vi "Stop Core.vi"(10 "final error code":i32, 11 "Car Wash Controller in":refnum<class "Car Wash Controller.lvclass">) -> (3 "Car Wash Controller out":refnum<class "Car Wash Controller.lvclass">)   [LabVIEW 2019, in "Car Wash Controller.lvlib" / "Car Wash Controller.lvclass"]
doc: "(<B>Filename</B>: Actor Framework.lvlib:Actor.lvclass:Stop Core.vi)\n\nDefines what the actor does before it stops. Use the <B>final error code</B> input to determine whether the actor shut down in response to an error.\n\nBy default, this method passes the Stop message along to all auto-stop nested actors. A descendant class may override this method to define additional behavior, such as shutting down any processes the actor initiated in its override of the Actor Core method."
uses:
  Car Wash Controller.lvclass
  Car Wash Controller.lvclass/Car Wash Controller.ctl
  <vilib>/ActorFramework/Actor/Actor.lvclass
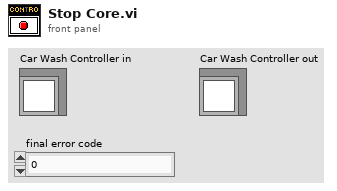
[diagram p1: front panel]
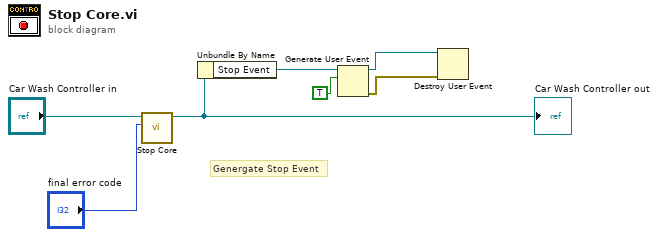
[diagram p0: block diagram]
diagram:
  # "Genergate Stop Event"
  n1 = call-parent "Stop Core.vi"("final error code"="final error code", "Actor in"="Car Wash Controller in") -> ("Actor out"=w5:refnum<class "Car Wash Controller.lvclass">)  [unwired: 9 in]
  "Car Wash Controller out" <- w5
  n2 = Unbundle By Name(w5) -> ("Stop Event"=w4:refnum<user-event>)
  n3 = Generate User Event(user event=w4, event data cluster=TRUE ("event data")) -> (user event out=w2:refnum<user-event>, error out=w3:errorcluster)  [unwired: 2 in]
  n4 = Destroy User Event(user event=w2, error in=w3) -> ()  [unwired: 1 out]
